vi "Configure Data Format.vi"(8 "error in (no error)":errorcluster, 10 "Format (0: ASCII)":u32(ring) items=["ASCII", "IEEE Std. 754 Double Precision", "IEEE Std. 754 Single Precision"], 11 "VISA resource name":refnum<visa-resource-name>) -> (0 "error out":errorcluster, 3 "VISA resource name out":refnum<visa-resource-name>)   [LabVIEW 2015, in "Keithley DMM6500 DAQ6500 Series.lvlib"]
doc: "Sets the data format that is used when transferring readings over the remote interface."
uses:
  <instrlib>/Keithley DMM6500 DAQ6500 Series/Keithley DMM6500 DAQ6500 Series.lvlib
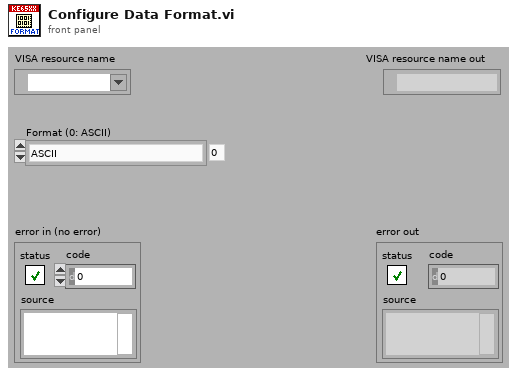
[diagram p1: front panel]
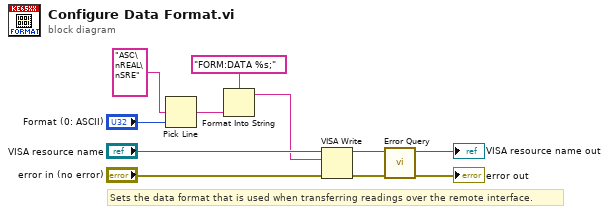
[diagram p0: block diagram]
diagram:
  # "Sets the data format that is used when transferring readings over the remote interface."
  n1 = Pick Line(multi-line string="ASC\nREAL\nSRE", line index="Format (0: ASCII)") -> (output string=w3:string)  [unwired: 1 in]
  n2 = Format Into String(format string="FORM:DATA %s;", w3) -> (resulting string=w5:string)  [unwired: 2 in, 1 out]
  n3 = VISA Write(VISA resource name="VISA resource name", write buffer=w5, error in (no error)="error in (no error)") -> (VISA resource name out=w9:refnum<visa-resource-name>, error out=w8:errorcluster)  [unwired: 1 out]
  n4 = call <instrlib>:"Error Query.vi"("error in (no error)"=w8, "VISA resource name"=w9) -> ("error out"=→"error out":errorcluster, "VISA resource name out"=→"VISA resource name out":refnum<visa-resource-name>)  [unwired: 6 in, 2 out]
